vi "Elevator - State Entry.vi"(8 "error in (no error)":errorcluster, 11 "View Model":T1) -> (0 "error out":errorcluster, 3 "View Model":T1)   [LabVIEW 2017]
doc: "Initializes state information at beginning of transition"
uses:
  View Model/Controls/View Model.ctl
  Configuration/Controls/Config Model.ctl
  Configuration/Controls/Config Data.ctl
  Error Handler/Controls/Error Model.ctl
  Error Handler/Controls/Error Data.ctl
  Error Handler/Controls/Error Type.ctl
  View Model/Controls/Shared Model.ctl
  Controls/Elevator Model.ctl
  Controls/Elevator Location.ctl
  Controls/Elevator CMD Data.ctl
  Controls/Elevator Commands.ctl
  Controls/Elevator Overhead.ctl
  Controls/Elevator States.ctl
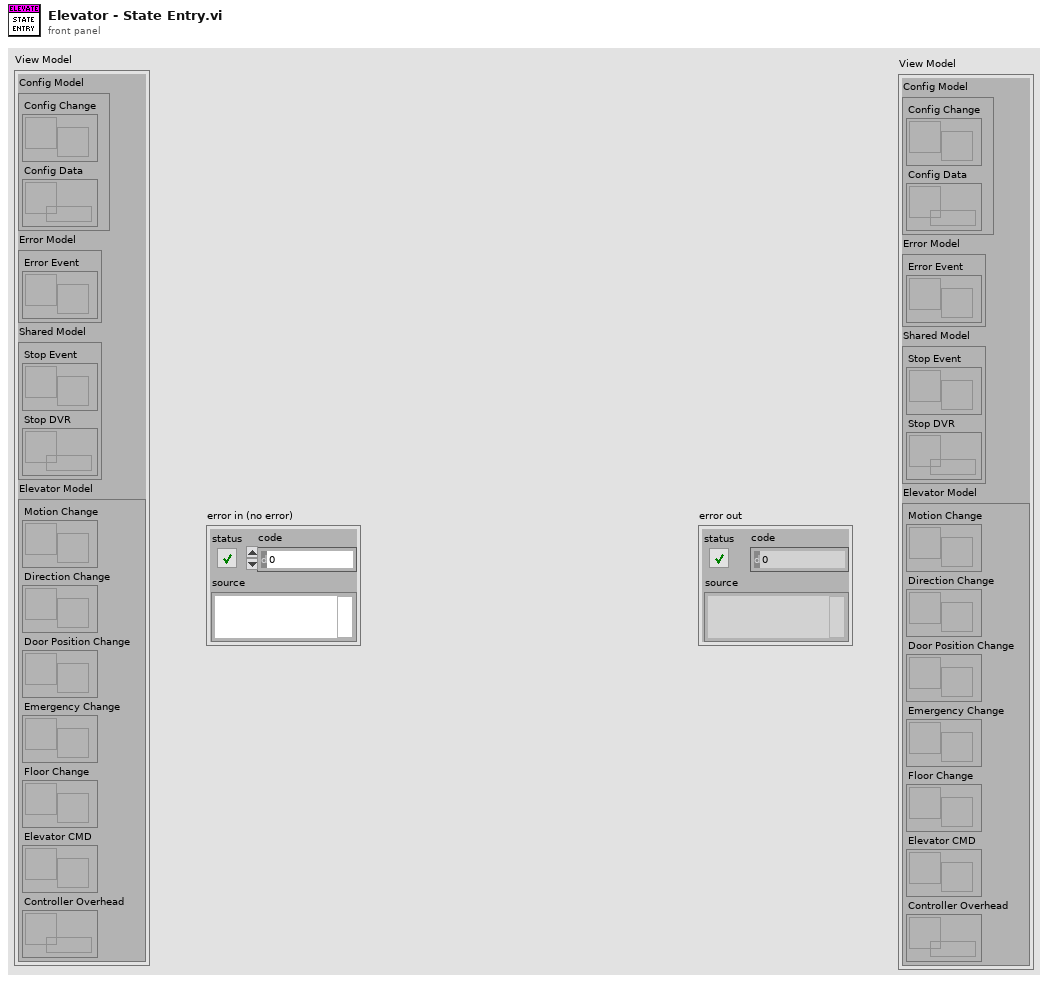
[diagram p1: front panel]
types:
  T1 = typedef "View Model.ctl" = cluster{"Config Model":T2, "Error Model":T3, "Shared Model":T4, "Elevator Model":T5}
  T2 = typedef "Config Model.ctl" = cluster{"Config Change":refnum<user-event>, "Config Data":refnum<data-value>}
  T3 = typedef "Error Model.ctl" = cluster{"Error Event":refnum<user-event>}
  T4 = typedef "Shared Model.ctl" = cluster{"Stop Event":refnum<user-event>, "Stop DVR":refnum<data-value>}
  T5 = typedef "Elevator Model.ctl" = cluster{"Motion Change":refnum<user-event>, "Direction Change":refnum<user-event>, "Door Position Change":refnum<user-event>, "Emergency Change":refnum<user-event>, "Floor Change":refnum<user-event>, "Elevator CMD":refnum<user-event>, "Controller Overhead":refnum<data-value>}
  T6 = typedef "Elevator States.ctl" = enum16{"Idle", "Init", "Open Doors", "Close Doors", "Start Move", "Move", "Finish Move", "Emergency", "Analysis", "Terminate"}
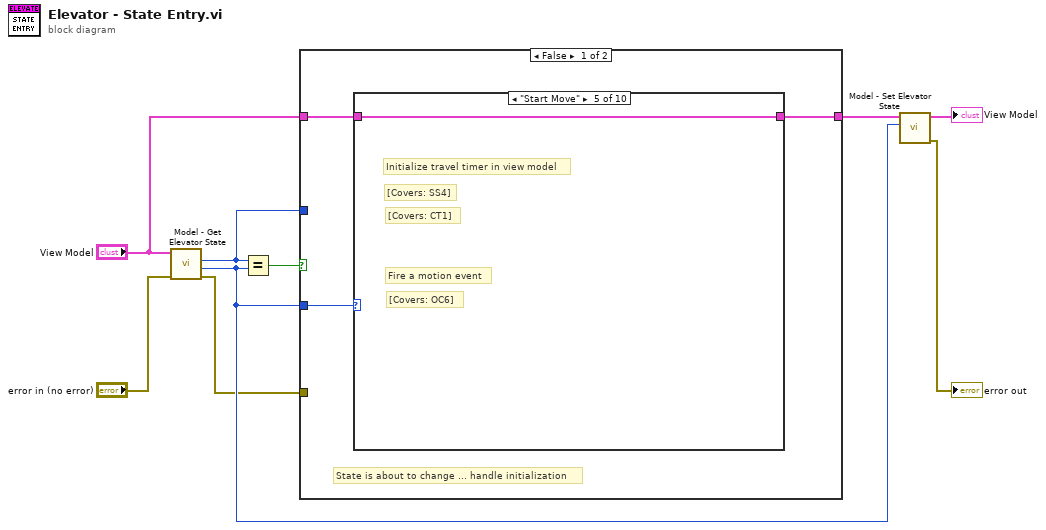
[diagram p0: block diagram]
diagram:
  n1 = call "Model - Get Elevator State.vi"("error in (no error)"="error in (no error)", "View Model"="View Model") -> ("error out"=w1:errorcluster, "Next Elevator State"=w4:T6, "Elevator State"=w6:T6)  [unwired: 6 in, 1 out]
  n2 = Equal?(x=w6, y=w4) -> (x = y?=w7:bool)
  n3 = case shown="False" w7 {
    tunnel: "View Model" -> [w12 w23]
    tunnel: w6 -> [_ _]
    tunnel: w4 -> [w10 _]
    tunnel: [w11 w23] -> w5
    tunnel: w1 -> [_ _]
    frame False {
      # "State is about to change ... handle initialization"
      n4 = case shown="\"Start Move\"" w10 {
        tunnel: w12 -> [w13 w14 w15 w16 w17 w18 w19 w20 w21 w22]
        tunnel: [w13 w14 w15 w16 w17 w18 w19 w20 w21 w22] -> w11
        frame "Idle", Default {
        }
        frame "Init" {
        }
        frame "Open Doors" {
          # "[Covers: OC3A]"
          # "[Covers: OC3]"
          # "Start open door timer"
        }
        frame "Close Doors" {
        }
        frame "Start Move" {
          # "[Covers: OC6]"
          # "Fire a motion event"
          # "[Covers: CT1]"
          # "[Covers: SS4]"
          # "Initialize travel timer in view model"
        }
        frame "Move" {
        }
        frame "Finish Move" {
        }
        frame "Emergency" {
        }
        frame "Analysis" {
        }
        frame "Terminate" {
        }
      }
    }
    frame True {
    }
  }
  n5 = call "Model - Set Elevator State.vi"("Elevator State"=w4, "View Model"=w5) -> ("error out"=→"error out":errorcluster, "View Model"=→"View Model":T1)  [unwired: 8 in]
